vi "configureTiming.vi"(8 "error in (no error)":errorcluster, 11 "AndorIKonAcquisitor in":refnum<class "AndorIKonAcquisitor.lvclass">) -> (0 "error out":errorcluster, 3 "AndorIKonAcquisitor out":refnum<class "AndorIKonAcquisitor.lvclass">)   [LabVIEW 2009, in "Hardware.lvlib" / "Channels.lvlib" / "AndorIKonAcquisitor.lvclass"]
uses:
  AndorIKonAcquisitor.lvclass
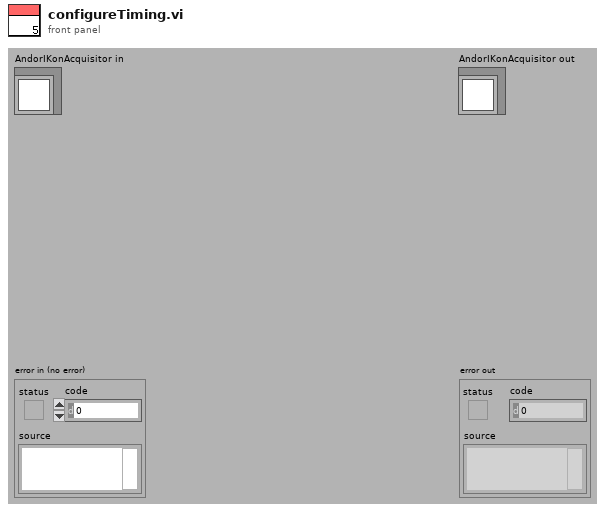
[diagram p1: front panel]
types:
  T1 = cluster{"shutter Open Time":dbl, "Shutter Close Time":dbl, "Exposure Time":dbl, " AccumulatedCycleTime":dbl, " KineticCycleTime":dbl, "Number of Accumulations":dbl, "Number in Kinetic Series ":dbl, "Shutter Mode":dbl}
  T2 = cluster{"Acquisition mode":dbl, "Readout Mode":dbl, "Gain":dbl}
  T3 = cluster{"Vertical Binning":dbl, "Horizontal Binning":dbl, "SubArea Height":dbl, "SubAreaWidth":dbl, "Offset":dbl, "Number of Tracks":dbl, "Track Positions":cluster{"Top":dbl, "Bottom ":dbl}[], "subArea Coordinate":dbl[]}
  T4 = cluster{"Vertical Shift Speed":dbl, "Horizontal Shift Speed":dbl, "Fast Kinetic V Shift Speed":dbl}
  T5 = cluster{"Vertical Shift Speeds":dbl[], "Horizontal Shift Speeds":dbl[]}
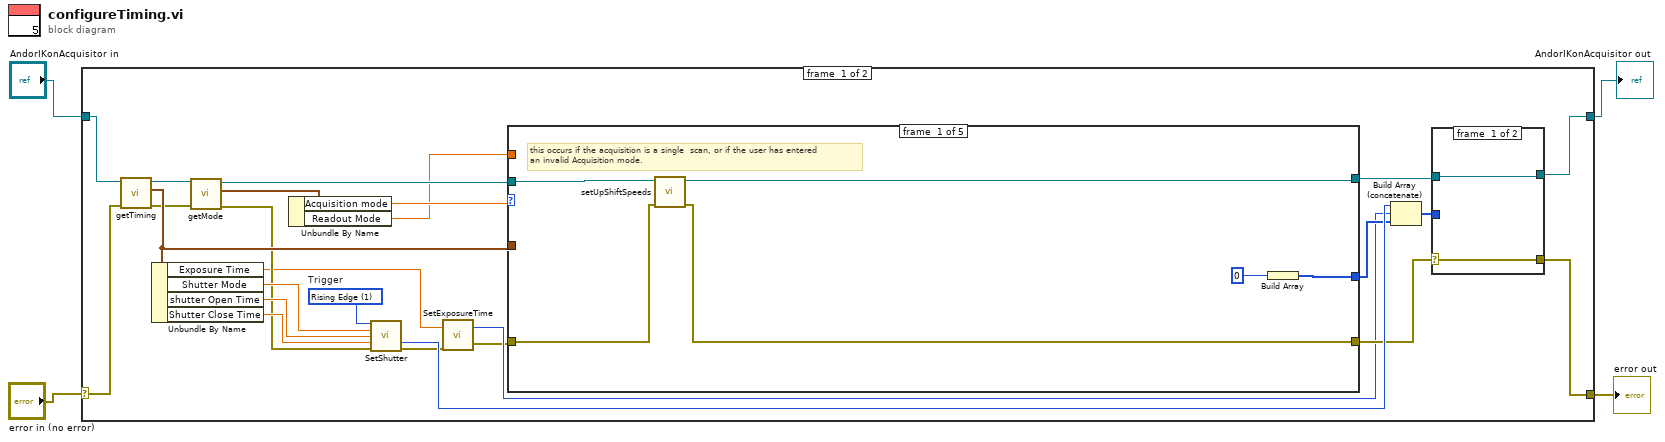
[diagram p0: block diagram]
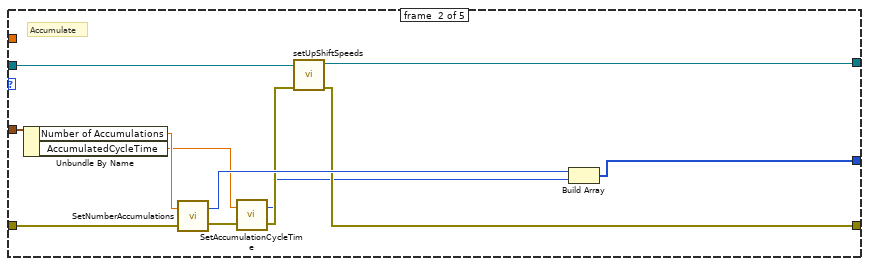
[diagram p2: hidden frame]
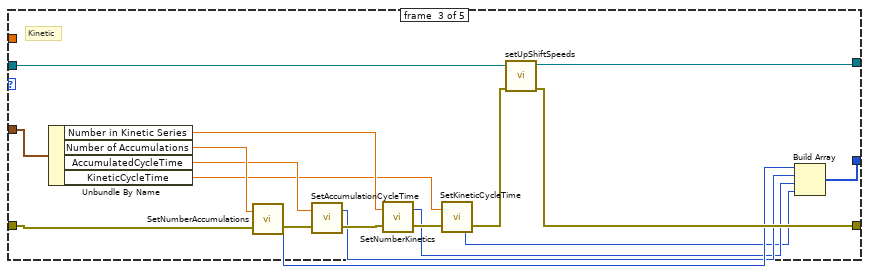
[diagram p3: hidden frame]
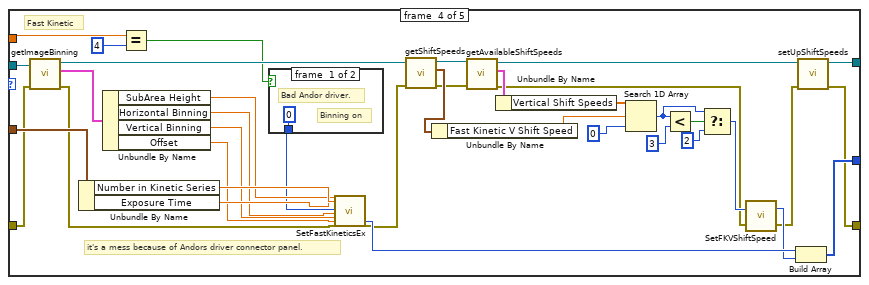
[diagram p4: hidden frame]
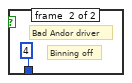
[diagram p5: hidden frame]
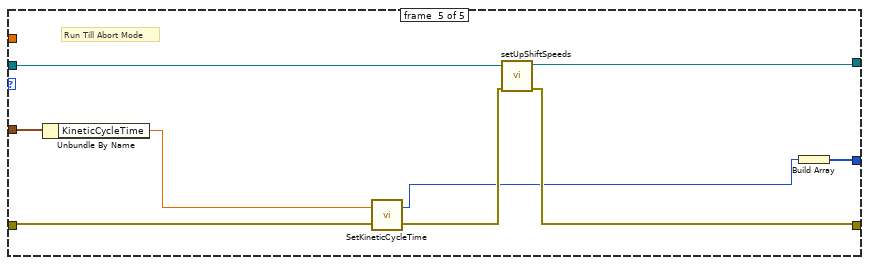
[diagram p6: hidden frame]
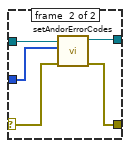
[diagram p7: hidden frame]
diagram:
  n1 = case shown="No Error" "error in (no error)" {
    selector: "error in (no error)" -> [w28 w122]
    tunnel: [w25 w122] -> w3
    tunnel: [w24 w121] -> w1
    tunnel: "AndorIKonAcquisitor in" -> [w29 w121]
    frame #0 {
      w23 = 1 items=["Rising Edge"=1, "Falling Edge"=0]  # Trigger
      n2 = call-dynamic "getTiming.vi"("error in (no error)"=w28, "CameraAcquisitor.lvclass in"=w29) -> ("error out"=w16:errorcluster, "Timing"=w17:T1, "CameraAcquisitor.lvclass out"=w18:refnum<class "AndorIKonAcquisitor.lvclass">)  [unwired: 7 in]
      n3 = Unbundle By Name(w17) -> ("Exposure Time"=w9:dbl, "Shutter Mode"=w19:dbl, "shutter Open Time"=w22:dbl, "Shutter Close Time"=w21:dbl)
      n4 = call-dynamic "getMode.vi"("error in (no error)"=w16, "CameraAcquisitor.lvclass in"=w18) -> ("error out"=w15:errorcluster, "Mode"=w14:T2, "CameraAcquisitor.lvclass out"=w6:refnum<class "AndorIKonAcquisitor.lvclass">)  [unwired: 7 in]
      n5 = Unbundle By Name(w14) -> ("Acquisition mode"=w11:dbl, "Readout Mode"=w5:dbl)
      n6 = call <userlib>:"SetShutter.vi"("type"=w23, "mode"=w19, "closingtime"=w22, "openingtime"=w21, "error in (no error)"=w15) -> ("DLL error code"=w26:u32, "error out"=w10:errorcluster)  [unwired: 9 in]
      n7 = call <userlib>:"SetExposureTime.vi"("error in (no error)"=w10, "time"=w9) -> ("error out"=w7:errorcluster, "DLL error code"=w8:u32)
      n8 = case shown="4" w11 {
        tunnel: w7 -> [w34 w47 w57 w99 w113]
        tunnel: [w33 w40 w60 w72 w108] -> w20
        tunnel: w17 -> [_ w46 w65 w102 w112]
        tunnel: [w32 w41 w61 w69 w107] -> w13
        tunnel: [w31 w44 w63 w90 w106] -> w12
        tunnel: w6 -> [w35 w42 w62 w87 w110]
        tunnel: w5 -> [_ _ _ w68 _]
        frame #0 {
          # "this occurs if the acquisition is a single  scan, or if the user has entered\nan invalid Acquisition mode."
          n9 = call "setUpShiftSpeeds.vi"("error in (no error)"=w34, "AndorIKonAcquisitor in"=w35) -> ("error out"=w33:errorcluster, "AndorIKonAcquisitor out"=w32:refnum<class "AndorIKonAcquisitor.lvclass">)  [unwired: 8 in]
          n10 = Build Array(0) -> (w31:i32[])
        }
        frame #1 {
          # "Accumulate"
          n11 = Unbundle By Name(w46) -> ("Number of Accumulations"=w45:dbl, "AccumulatedCycleTime"=w37:dbl)
          n12 = call <userlib>:"SetNumberAccumulations.vi"("error in (no error)"=w47, "number"=w45) -> ("error out"=w39:errorcluster, "DLL error code"=w43:u32)
          n13 = call <userlib>:"SetAccumulationCycleTime.vi"("error in (no error)"=w39, "time"=w37) -> ("error out"=w38:errorcluster, "DLL error code"=w36:u32)
          n14 = call "setUpShiftSpeeds.vi"("error in (no error)"=w38, "AndorIKonAcquisitor in"=w42) -> ("error out"=w40:errorcluster, "AndorIKonAcquisitor out"=w41:refnum<class "AndorIKonAcquisitor.lvclass">)  [unwired: 8 in]
          n15 = Build Array(w43, w36) -> (w44:u32[])
        }
        frame #2 {
          # "Kinetic"
          n16 = Unbundle By Name(w65) -> ("Number in Kinetic Series"=w64:dbl, "Number of Accumulations"=w56:dbl, "AccumulatedCycleTime"=w55:dbl, "KineticCycleTime"=w53:dbl)
          n17 = call <userlib>:"SetNumberAccumulations.vi"("error in (no error)"=w57, "number"=w56) -> ("error out"=w59:errorcluster, "DLL error code"=w51:u32)
          n18 = call <userlib>:"SetAccumulationCycleTime.vi"("error in (no error)"=w59, "time"=w55) -> ("error out"=w58:errorcluster, "DLL error code"=w50:u32)
          n19 = call <userlib>:"SetNumberKinetics.vi"("error in (no error)"=w58, "number"=w64) -> ("error out"=w54:errorcluster, "DLL error code"=w49:u32)
          n20 = call <userlib>:"SetKineticCycleTime.vi"("error in (no error)"=w54, "time"=w53) -> ("error out"=w52:errorcluster, "DLL error code"=w48:u32)
          n21 = call "setUpShiftSpeeds.vi"("error in (no error)"=w52, "AndorIKonAcquisitor in"=w62) -> ("error out"=w60:errorcluster, "AndorIKonAcquisitor out"=w61:refnum<class "AndorIKonAcquisitor.lvclass">)  [unwired: 8 in]
          n22 = Build Array(w51, w50, w49, w48) -> (w63:u32[])
        }
        frame #3 {
          # "it's a mess because of Andors driver connector panel."
          # "Fast Kinetic"
          n23 = call-dynamic "getImageBinning.vi"("error in (no error)"=w99, "CameraAcquisitor.lvclass in"=w87) -> ("error out"=w97:errorcluster, "Image Binning"=w98:T3, "CameraAcquisitor.lvclass out"=w89:refnum<class "AndorIKonAcquisitor.lvclass">)  [unwired: 7 in]
          n24 = Unbundle By Name(w102) -> ("Number in Kinetic Series"=w101:dbl, "Exposure Time"=w100:dbl)
          n25 = Unbundle By Name(w98) -> ("SubArea Height"=w96:dbl, "Horizontal Binning"=w94:dbl, "Vertical Binning"=w93:dbl, "Offset"=w92:dbl)
          n26 = Equal?(x=w68, y=4) -> (x = y?=w66:bool)
          n27 = case shown="True" w66 {
            tunnel: [0 4] -> w95
            frame #0 {
              # "Binning on"
              # "Bad Andor driver."
            }
            frame #1 {
              # "Binning off"
              # "Bad Andor driver"
            }
          }
          n28 = call <userlib>:"SetFastKineticsEx.vi"("height"=w96, "series"=w101, "exptime"=w100, "mode"=w95, "hbin (1)"=w94, "vbin (1)"=w93, "offset"=w92, "error in (no error)"=w97) -> ("DLL error code"=w91:u32, "error out"=w86:errorcluster)  [unwired: 18 in]
          n29 = call-dynamic "getShiftSpeeds.vi"("error in (no error)"=w86, "CameraAcquisitor.lvclass in"=w89) -> ("error out"=w74:errorcluster, "Shift Speed"=w88:T4, "CameraAcquisitor.lvclass out"=w85:refnum<class "AndorIKonAcquisitor.lvclass">)  [unwired: 7 in]
          n30 = Unbundle By Name(w88) -> ("Fast Kinetic V Shift Speed"=w82:dbl)
          n31 = call "getAvailableShiftSpeeds.vi"("error in (no error)"=w74, "AndorIKonAcquisitor.lvclass in"=w85) -> ("error out"=w73:errorcluster, "Available Shift Speeds"=w84:T5, "AndorIKonAcquisitor.lvclass out"=w75:refnum<class "AndorIKonAcquisitor.lvclass">)  [unwired: 7 in]
          n32 = Unbundle By Name(w84) -> ("Vertical Shift Speeds"=w83:dbl[])
          n33 = Search 1D Array(1D array=w83, element=w82, start index (0)=0) -> (index of element=w78:i32)
          n34 = Less?(x=w78, y=3) -> (x < y?=w79:bool)
          n35 = Select(t=w78, s=w79, f=2) -> (s? t:f=w76:i32)
          n36 = call <userlib>:"SetFKVShiftSpeed.vi"("error in (no error)"=w73, "index"=w76) -> ("error out"=w70:errorcluster, "DLL error code"=w71:u32)
          n37 = Build Array(w91, w71) -> (w90:u32[])
          n38 = call "setUpShiftSpeeds.vi"("error in (no error)"=w70, "AndorIKonAcquisitor in"=w75) -> ("error out"=w72:errorcluster, "AndorIKonAcquisitor out"=w69:refnum<class "AndorIKonAcquisitor.lvclass">)  [unwired: 8 in]
        }
        frame #4 {
          # "Run Till Abort Mode"
          n39 = Unbundle By Name(w112) -> ("KineticCycleTime"=w111:dbl)
          n40 = call <userlib>:"SetKineticCycleTime.vi"("error in (no error)"=w113, "time"=w111) -> ("error out"=w109:errorcluster, "DLL error code"=w105:u32)
          n41 = call "setUpShiftSpeeds.vi"("error in (no error)"=w109, "AndorIKonAcquisitor in"=w110) -> ("error out"=w108:errorcluster, "AndorIKonAcquisitor out"=w107:refnum<class "AndorIKonAcquisitor.lvclass">)  [unwired: 8 in]
          n42 = Build Array(w105) -> (w106:u32[])
        }
      }
      n43 = Build Array (concatenate)(w26, w8, w12) -> (w27:u32[])
      n44 = case shown="Error" w20 {
        selector: w20 -> [w115 w120]
        tunnel: w13 -> [w114 w116]
        tunnel: [w114 w118] -> w24
        tunnel: [w115 w119] -> w25
        tunnel: w27 -> [_ w117]
        frame #0 {
        }
        frame #1 {
          n45 = call-dynamic "setAndorErrorCodes.vi"("error in (no error)"=w120, "Andor Error Codes"=w117, "AndorIKonAcquisitor.lvclass in"=w116) -> ("error out"=w119:errorcluster, "AndorIKonAcquisitor.lvclass out"=w118:refnum<class "AndorIKonAcquisitor.lvclass">)  [unwired: 7 in]
        }
      }
    }
    frame #1 {
    }
  }
  "error out" <- w3
  "AndorIKonAcquisitor out" <- w1
